vi "CHECK OUT ITEM LOCATION VALUE UPDATE.vi"(10 "Location Selection String":refnum<vi>, 11 "Items Listbox":refnum<vi>) -> ()   [LabVIEW 2019]
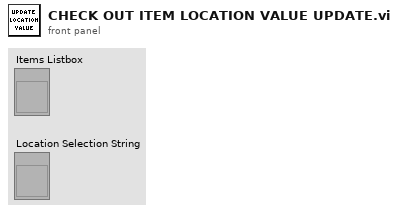
[diagram p1: front panel]
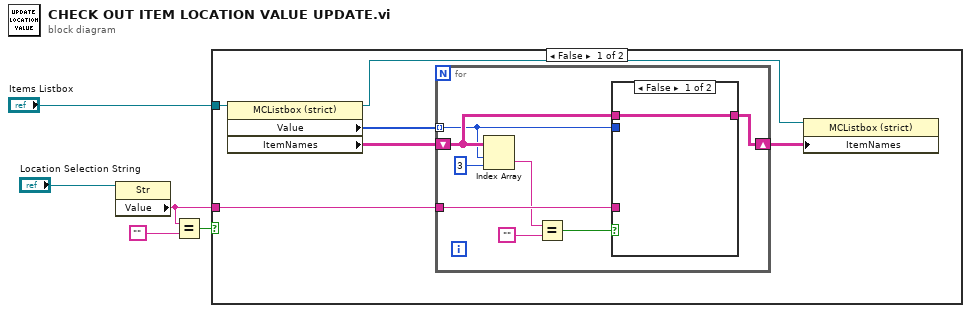
[diagram p0: block diagram]
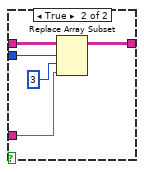
[diagram p2: hidden frame]
diagram:
  n1 = property class="Str"(reference="Location Selection String") -> ("Value"=w1:string)  [unwired: 1 in, 2 out]
  n2 = Equal?(x=w1, y="") -> (x = y?=w2:bool)
  n3 = case shown="False" w2 {
    tunnel: "Items Listbox" -> [w11 _]
    tunnel: w1 -> [w8 _]
    frame False {
      n4 = property class="MCListbox (strict)"(reference=w11) -> (reference out=w7:refnum<vi>, "Value"=w10:i32[], "ItemNames"=w9:string[][])  [unwired: 1 in, 1 out]
      n5 = for {
        tunnel: w10 -> [w13] mode=indexing
        tunnel: w8 -> [w16]
        shift-right: [w12] -> w6
        shift-left: w9 -> [w14]
        n6 = Index Array(array=w14, index (row)=w13, index (col)=3 ("disabled index (col)")) -> (element=w15:string)
        n7 = Equal?(x=w15, y="") -> (x = y?=w17:bool)
        n8 = case shown="False" w17 {
          tunnel: w16 -> [_ w22]
          tunnel: w14 -> [w20 w25]
          tunnel: w13 -> [_ w24]
          tunnel: [w20 w21] -> w12
          frame False {
          }
          frame True {
            n9 = Replace Array Subset(array=w25, new element=w22, index (row)=w24, index (col)=3 ("disabled index (col)")) -> (w21:string[][])
          }
        }
      }
      n10 = property class="MCListbox (strict)"(reference=w7, "ItemNames"=w6) -> ()  [unwired: 1 in, 2 out]
    }
    frame True {
    }
  }
